vi "ABB hasp ErrorLookup.vi"(3 "ReturnVal":i16) -> (0 "error out":errorcluster)   [LabVIEW 2017]
panel:
  in  "Code":i32[](array[numeric])=[0, -999, -121, -120, -112, -111, -110, -102, -101, -100, -29, -28, -27, -26, -25, -24, -23, -22, -21, -20, -13, -12, -11, -10, -9, -8, -7, -6, -5, -4, -3, -3, -2, -1, 1, 2, 3, 4, 5, 6, 7, 8, 10, 11, 15, 18, 19, 20, 21, 22, 23, 24, 25, 26, 28, 30, 33, 40, 129, 130, 131, 132, 133, 134, 135, 136, 137, 138, 139, 140, 141, 142, 150, 152, 153, 155, 157, 0]
  in  "Message":string[][](array[string])=[[" 0", " Operation successful                                                           */"], ["-999", " HASP Invalid Service                                                           */"], ["-121", " Cannot free DOS Memory                                                         */"], ["-120", " Cannot allocate DOS Memory                                                     */"], ["-112", " Cannot close the HASP Device Driver                                            */"], ["-111", " Cannot read the HASP Device Driver                                             */"], ["-110", " Cannot open the HASP Device Driver                                             */"], ["-102", " Cannot close the HASP Device Driver                                            */"], ["-101", " Cannot read the HASP Device Driver                                             */"], ["-100", " Cannot open the HASP Device Driver                                             */"], ["-29", " A HASP was found but it is not a TimeHASP                                      */"], ["-28", " A HASP with specified passwords was not found                                  */"], ["-27", " Timeout - Write operation failed                                               */"], ["-26", " Invalid address - Address is not in 0 - 15                                     */"], ["-25", " Invalid Hour                                                                   */"], ["-24", " Invalid Minute                                                                 */"], ["-23", " Invalid Second                                                                 */"], ["-22", " Invalid year                                                                   */"], ["-21", " Invalid month                                                                  */"], ["-20", " Invalid day                                                                    */"], ["-13", " Driver version mismatch                                                        */"], ["-12", " Invalid parameter                                                              */"], ["-11", " Terminal Server under SP3 is not supported                                     */"], ["-10", " Terminal Server was found.                                                     */"], ["-9", " Invalid pointer used by Encode Data                                            */"], ["-8", " The hardware does not support the service                                      */"], ["-7", " The data length is too short                                                   */"], ["-6", " Parallel port is busy.                                                         */"], ["-5", " Unsuccessful Write operation                                                   */"], ["-4", " A HASP was found but it is not a MemoHASP                                      */"], ["-3", " A HASP with specified passwords was not found                                  */"], ["-3", " A HASP with specified passwords was not found                                  */"], ["-2", " Address out of range                                                           */"], ["-1", " Timeout - Write operation failed                                               */"], ["1", " IPX, NetBIOS, or TCP/IP protocols have not been installed properly.            */"], ["2", " Communication Error - unable to get the socket number (TCP/IP, IPX)            */"], ["3", " Communication Error.                                                           */"], ["4", " No NetHASP License Manager was found.                                          */"], ["5", " Cannot read NetHASP License Manager address file                               */"], ["6", " Cannot close NetHASP License Manager address file                              */"], ["7", " Communication error - failed to send packet (IPX, NetBIOS                      */"], ["8", " No answer from the NetHASP License Manager.                                    */"], ["10", " Service requested before LOGIN                                                 */"], ["11", " NetBIOS: Communication error - adapter error                                   */"], ["15", " No active NetHASP Licence Manager was found                                    */"], ["18", " Cannot perform LOGIN - SetServerByName failed                                  */"], ["19", " NetHASP configuration file syntax error                                        */"], ["20", " Error handling NetHASP configuration file                                      */"], ["21", " Memory allocation error                                                        */"], ["22", " Memory release error                                                           */"], ["23", " Invalid NetHASP memory address                                                 */"], ["24", " Error trying to Encrypt/Decrypt                                                */"], ["25", " TCP/IP: failed to load WINSOCK.DLL                                             */"], ["26", " TCP/IP: failed to unload WINSOCK.DLL                                           */"], ["28", " TCP/IP: WINSOCK.DLL startup error                                              */"], ["30", " TCP/IP: Failed to close socket.                                                */"], ["33", " SetProtocol service requested without performing LOGOUT                        */"], ["40", " NetHASP services are not supported                                             */"], ["129", " NetHASP key is not connected to the NetHASP Licence Manager                    */"], ["130", " Program Number is not in the Program List of the NetHASP memory                */"], ["131", " Error reading NetHASP memory                                                   */"], ["132", " Error writing NetHASP memory                                                   */"], ["133", " Number of stations exceeded                                                    */"], ["134", " Number of activations exceeded                                                 */"], ["135", " LOGOUT called without LOGIN                                                    */"], ["136", " NetHASP Licence Manager is busy                                                */"], ["137", " No space in NetHASP Log Table                                                  */"], ["138", " NetHASP Internal error                                                         */"], ["139", " NetHASP Licence Manager crashed and reactivated                                */"], ["140", " NetHASP Licence Manager does not support the station's network                 */"], ["141", " Invalid Service NetHASP Licence Manager does not support the station's network */"], ["142", " Invalid NetHASP Licence Manager name in configuration file                     */"], ["150", " Invalid NetHASP Licence Manager name in SetServerByName                        */"], ["152", " Error trying to encrypt by the LM                                              */"], ["153", " Error trying to decrypt by the LM                                              */"], ["155", " LM old version was found                                                       */"], ["157            /* specified buffer size is too small for requested function                      */", " specified buffer size is too small for requested function                      */"], ["", ""]]
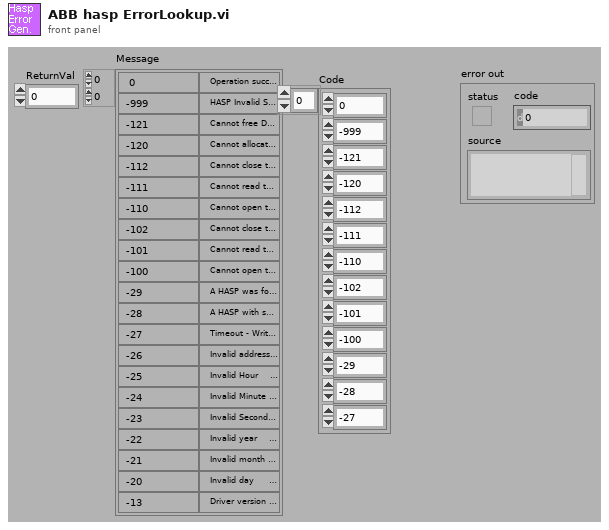
[diagram p1: front panel]
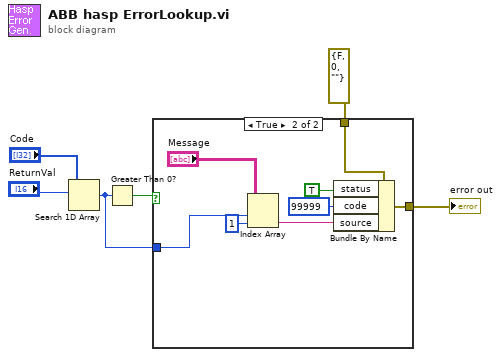
[diagram p0: block diagram]
diagram:
  n1 = Search 1D Array(1D array="Code", element="ReturnVal") -> (index of element=w3:i32)  [unwired: 1 in]
  n2 = Greater Than 0?(x=w3) -> (x > 0?=w4:bool)
  n3 = case shown="True" w4 {
    tunnel: w3 -> [_ w11]
    tunnel: errorcluster {"status"=FALSE, "code"=0, "source"=""} ("error out") -> [w7 w13]
    tunnel: [w7 w9] -> w1
    frame False {
    }
    frame True {
      n4 = Index Array(array="Message", index (row)=w11, index (col)=1 ("disabled index (col)")) -> (element=w10:string)
      n5 = Bundle By Name(cluster=w13, "status"=TRUE, "code"=99999, "source"=w10) -> (w9:errorcluster)
    }
  }
  "error out" <- w1
